vi "Alicat set.vi"(10 "Byte array":u8[](array[numeric])=[65, 48, 48, 48, 48, 48, 13, 68, 48, 48, 48, 48, 48, 13, 69, 48, 48, 48, 48, 48, 13, 70, 48, 48, 48, 48, 48, 0]) -> ()   [LabVIEW 2014]
uses:
  <vilib>/eio/EIOMethodNode/EIOMethodNode.xnode
  <vilib>/rvi/eio/common/nirviEmuTemplateMethod_errors.vi
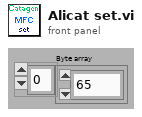
[diagram p1: front panel]
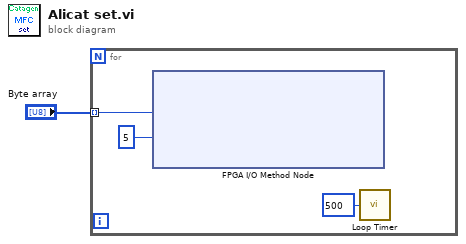
[diagram p0: block diagram]
diagram:
  n1 = for {
    tunnel: "Byte array" -> [w3] mode=indexing
    n2 = xnode "FPGA I/O Method Node"("Data"=w3, "Timeout (ms)"=5) -> ()  [unwired: 2 in, 3 out]
    n3 = call "Loop Timer"("Count(uSec)"=u32 500) -> ()  [unwired: 1 out]
  }
